vi "ExpXpecParser.vi"() -> ()   [LabVIEW 2010]
uses:
  <vilib>/xml/NI_XML.lvlib
panel:
  out "error in (no error)":errorcluster
  out "CSG 2":csg caption="CSG"
  out "CDB 2":cdb caption="CDB"
  out "CXT 2":cxt caption="CXT"
  out "U 65":u64 caption="U 64"
  out "U 33":u32 caption="U 32"
  out "U 17":u16 caption="U 16"
  out "I 9":i64 caption="I 8"
  out "I 65":i64 caption="I 64"
  out "EXT 2":ext caption="EXT"
  out "I16 2":i16
  out "FXP 2":fxp<+,1,1> caption="FXP"
  out "Single 2":sgl
  out "I 33":i32 caption="I 32"
  out "U 9":i32 caption="U 8"
  out "String 2":string caption="String"
  out "Double 2":dbl caption="Double"
  out "parse errors":string
  in  "Root in":string="/experimentSpecification/terminal/function/"
  in  "input array":variant[](array[variant])
  out "XML-String-in":string
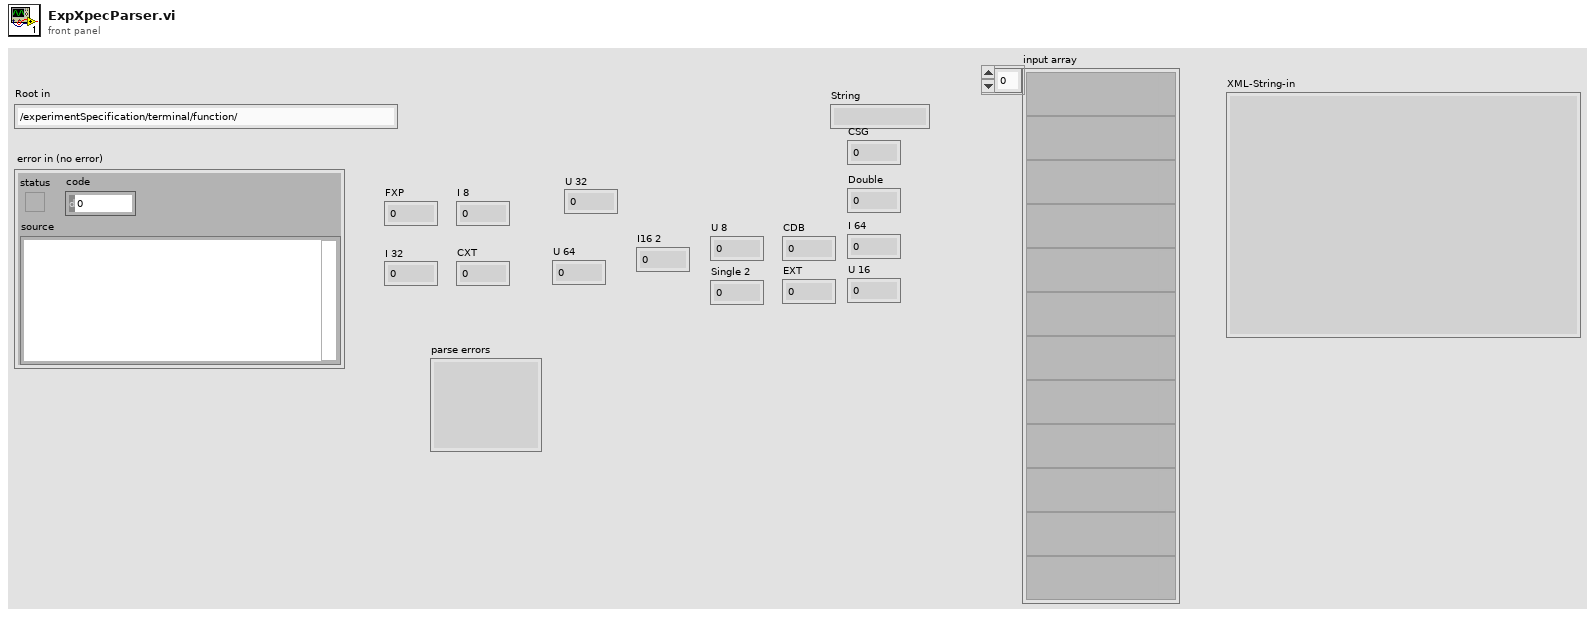
[diagram p1: front panel]
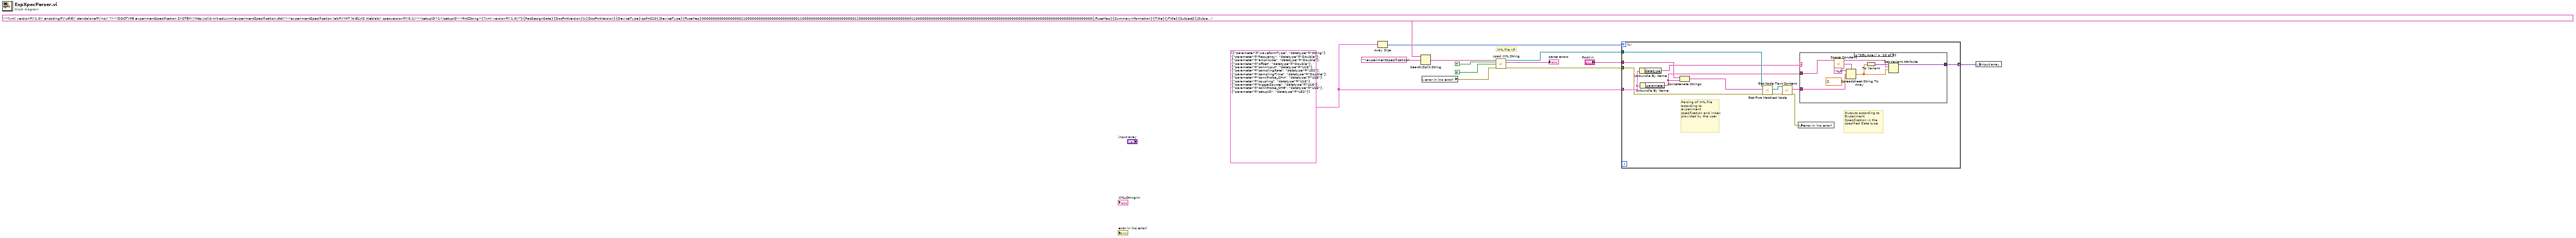
[diagram p0: block diagram]
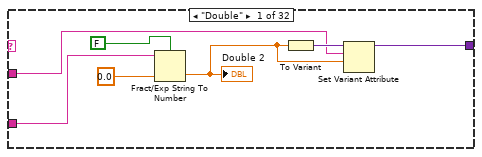
[diagram p2: hidden frame]
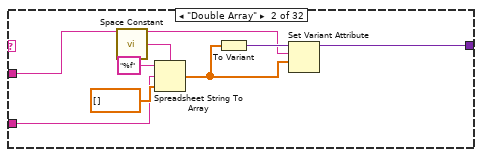
[diagram p3: hidden frame]
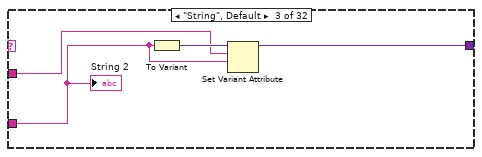
[diagram p4: hidden frame]
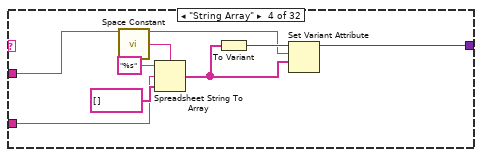
[diagram p5: hidden frame]
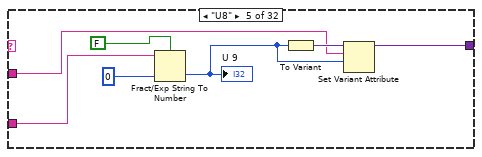
[diagram p6: hidden frame]
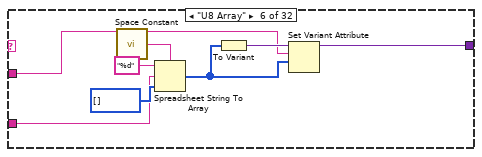
[diagram p7: hidden frame]
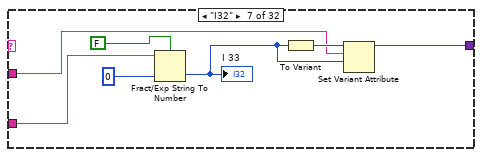
[diagram p8: hidden frame]
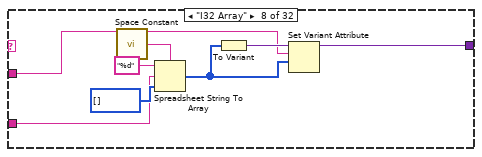
[diagram p9: hidden frame]
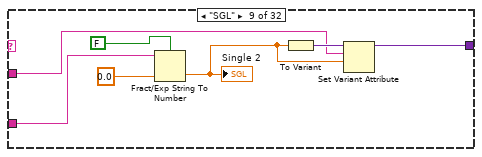
[diagram p10: hidden frame]
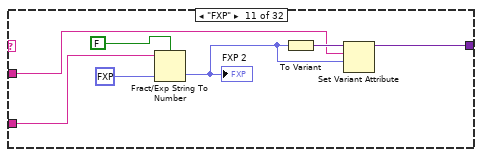
[diagram p11: hidden frame]
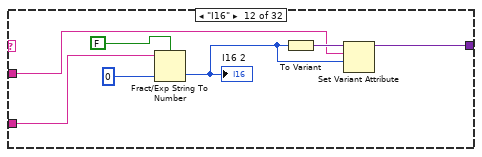
[diagram p12: hidden frame]
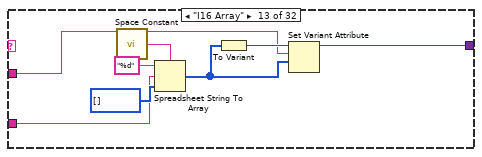
[diagram p13: hidden frame]
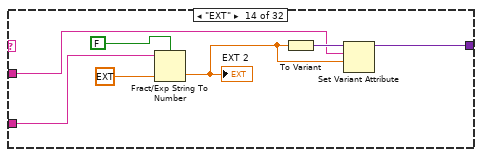
[diagram p14: hidden frame]
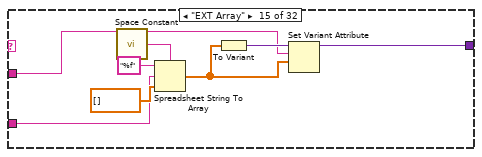
[diagram p15: hidden frame]
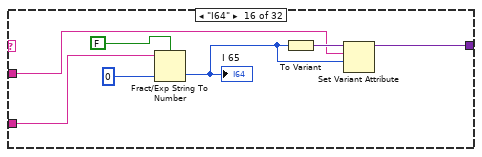
[diagram p16: hidden frame]
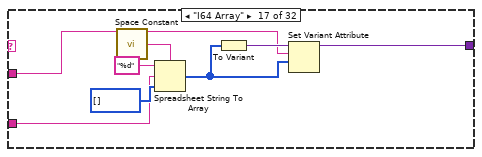
[diagram p17: hidden frame]
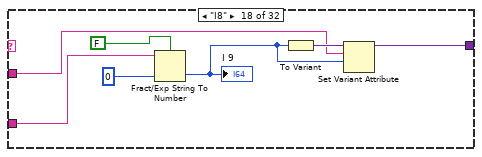
[diagram p18: hidden frame]
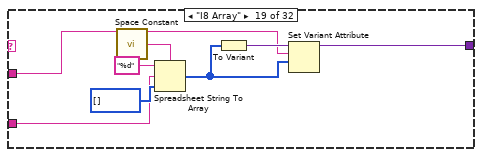
[diagram p19: hidden frame]
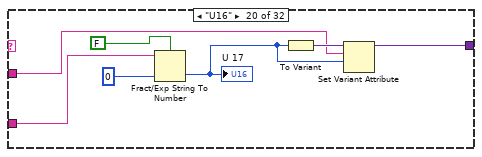
[diagram p20: hidden frame]
diagram:
  w3 = cluster{"parameter":string, "datatype":string}[] [{"parameter"="waveformType", "datatype"="String"}, {"parameter"="frequency", "datatype"="Double"}, {"parameter"="amplitude", "datatype"="Double"}, {"parameter"="offset", "datatype"="Double"}, {"parameter"="connInput", "datatype"="U16"}, {"parameter"="samplingRate", "datatype"="U32"}, {"parameter"="samplingTime", "datatype"="Double"}, {"parameter"="connProbe_CHA", "datatype"="U16"}, {"parameter"="coupling", "datatype"="U16"}, {"parameter"="triggerSource", "datatype"="U16"}, {"parameter"="connProbe_CHB", "datatype"="U16"}, {"parameter"="setupID", "datatype"="U32"}] ("Parameter in")
  # "XML file I/P"
  n1 = Array Size(array=w3) -> (size(s)=w1:i32)
  n2 = Search/Split String(string="<?xml version=\"1.0\" encoding=\"utf-8\" standalone=\"no\" ?><!DOCTYPE experimentSpecification SYSTEM \"http://olid.mit.edu/xml/experimentSpecification.dtd\"><experimentSpecification lab=\"MIT NI-ELVIS Weblab\" specversion=\"0.1\"><setupID>1</setupID><PACString>{?xml version=\"1.0\"?}{PacDesignData}{DocFmtVersion}1{/DocFmtVersion}{DeviceType}ispPAC10{/DeviceType}{FuseMap}00000000000000000011000000000000000000000000110000000000000000000000001100000000000000000000000011000000000000000000000000000000000000000000000000000000000000000000000000000000000{/FuseMap}{SummaryInformation}{Title}{/Title}{Subject}{/Subject}{Author}CTI{/Author}{Keywords}ispPAC10{/Keywords}{Comments}{![CDATA[]]}{/Comments}{/SummaryInformation}{/PacDesignData}</PACString><terminal instrumentType=\"FGEN\" instrumentNumber=\"1\"><vname download=\"true\">Vin</vname><function type=\"WAVEFORM\"><waveformType>SINE</waveformType><frequency>100.0</frequency><amplitude>1.0</amplitude><offset>5.0</offset><connInput>0</connInput></function></terminal><terminal instrumentType=\"SCOPE\" instrumentNumber=\"2\"><vname download=\"true\">Vout</vname><function type=\"SAMPLING\"><samplingRate>100000</samplingRate><samplingTime>0.01</samplingTime><connProbe_CHA>0</connProbe_CHA><coupling>1</coupling><triggerSource>0</triggerSource><connProbe_CHB>0</connProbe_CHB></function></terminal></experimentSpecification>" ("XML-String-in"), search string/char (-)="<experimentSpecification") -> (match + rest of string=w4:string)  [unwired: 1 in, 2 out]
  n3 = local read "error in (no error)"() -> (w6:errorcluster)
  n4 = call <vilib>:"Load XML String.vi"("XML string"=w4, "process namespaces (False)"=TRUE, "process schema (False)"=FALSE, "error in (no error)"=w6) -> ("DOM document out"=w9:refnum<k20>, "parse errors"=→"parse errors":string, "error out"=w10:errorcluster)  [unwired: 9 out]
  n5 = for {
    N: w1 -> [_]
    tunnel: w9 -> [w25]
    tunnel: "Root in" -> [w22]
    tunnel: w3 -> [w20] mode=indexing
    tunnel: w10 -> [w19]
    tunnel: [w18] -> w7 mode=indexing
    # "Outputs according to Experiment Specification in the specified Data type"
    # "Parsing of XML file according to experiment specification and index provided by the user"
    n6 = Unbundle By Name(w20) -> ("datatype"=w17:string)
    n7 = Unbundle By Name(w20) -> ("parameter"=w15:string)
    n8 = Concatenate Strings(w22, w15) -> (w21:string)
    n9 = call <vilib>:"Get First Matched Node.vi"("error in (no error)"=w19, "XPath expression"=w21, "node in"=w25) -> ("error out"=w23:errorcluster, "node result"=w24:refnum<k20>)  [unwired: 6 in, 1 out]
    n10 = call <vilib>:"Get Node Text Content.vi"("error in (no error)"=w23, "node in"=w24) -> ("error out"=w14:errorcluster, "node text"=w16:string)  [unwired: 7 in, 1 out]
    n11 = local write "error in (no error)"(w14) -> ()
    n12 = case shown="\"SGL Array\"" w17 {
      tunnel: w15 -> [w26 w34 w41 w45 w53 w60 w68 w76 w83 w91 w98 w105 w112 w120 w128 w135 w142 w150 w157 w165 w172 w180 w187 w195 w202 w210 w218 w226 w233 w240 w248 w255]
      tunnel: w16 -> [w27 w33 w42 w46 w54 w61 w69 w75 w84 w90 w99 w106 w113 w121 w127 w136 w143 w151 w158 w166 w173 w181 w188 w196 w203 w211 w217 w225 w232 w241 w247 w256]
      tunnel: [w29 w36 w43 w49 w56 w64 w71 w79 w86 w93 w101 w108 w116 w123 w130 w138 w146 w153 w161 w168 w176 w183 w191 w198 w206 w213 w220 w228 w235 w243 w250 w258] -> w18
      frame "Double" {
        n13 = Fract/Exp String To Number(use system decimal point (T)=FALSE, string=w27, default (0 dbl)=0.0) -> (number=w28:dbl)  [unwired: 1 in, 1 out]
        "Double 2" <- w28
        n14 = To Variant(anything=w28) -> (Variant=w30:variant)
        n15 = Set Variant Attribute(Variant=w30, name=w26, value=w28) -> (Variant out=w29:variant)  [unwired: 1 in, 2 out]
      }
      frame "Double Array" {
        n16 = call <vilib>:"Space Constant.vi"() -> ("String"=w38:string)
        n17 = Spreadsheet String To Array(delimiter (Tab)=w38, format string="%f", spreadsheet string=w33, array type (2D Dbl)=dbl[] [] ("Array")) -> (array=w35:dbl[])
        n18 = To Variant(anything=w35) -> (Variant=w37:variant)
        n19 = Set Variant Attribute(Variant=w37, name=w34, value=w35) -> (Variant out=w36:variant)  [unwired: 1 in, 2 out]
      }
      frame "String", Default {
        n20 = To Variant(anything=w42) -> (Variant=w44:variant)
        n21 = Set Variant Attribute(Variant=w44, name=w41, value=w42) -> (Variant out=w43:variant)  [unwired: 1 in, 2 out]
        "String 2" <- w42
      }
      frame "String Array" {
        n22 = call <vilib>:"Space Constant.vi"() -> ("String"=w51:string)
        n23 = Spreadsheet String To Array(delimiter (Tab)=w51, format string="%s", spreadsheet string=w46, array type (2D Dbl)=string[] [] ("Array")) -> (array=w48:string[])
        n24 = To Variant(anything=w48) -> (Variant=w50:variant)
        n25 = Set Variant Attribute(Variant=w50, name=w45, value=w48) -> (Variant out=w49:variant)  [unwired: 1 in, 2 out]
      }
      frame "U8" {
        n26 = Fract/Exp String To Number(use system decimal point (T)=FALSE, string=w54, default (0 dbl)=u8 0) -> (number=w55:u8)  [unwired: 1 in, 1 out]
        "U 9" <- w55
        n27 = To Variant(anything=w55) -> (Variant=w57:variant)
        n28 = Set Variant Attribute(Variant=w57, name=w53, value=w55) -> (Variant out=w56:variant)  [unwired: 1 in, 2 out]
      }
      frame "U8 Array" {
        n29 = call <vilib>:"Space Constant.vi"() -> ("String"=w66:string)
        n30 = Spreadsheet String To Array(delimiter (Tab)=w66, format string="%d", spreadsheet string=w61, array type (2D Dbl)=u8[] [] ("Array")) -> (array=w62:u8[])
        n31 = To Variant(anything=w62) -> (Variant=w65:variant)
        n32 = Set Variant Attribute(Variant=w65, name=w60, value=w62) -> (Variant out=w64:variant)  [unwired: 1 in, 2 out]
      }
      frame "I32" {
        n33 = Fract/Exp String To Number(use system decimal point (T)=FALSE, string=w69, default (0 dbl)=0) -> (number=w70:i32)  [unwired: 1 in, 1 out]
        "I 33" <- w70
        n34 = To Variant(anything=w70) -> (Variant=w72:variant)
        n35 = Set Variant Attribute(Variant=w72, name=w68, value=w70) -> (Variant out=w71:variant)  [unwired: 1 in, 2 out]
      }
      frame "I32 Array" {
        n36 = call <vilib>:"Space Constant.vi"() -> ("String"=w81:string)
        n37 = Spreadsheet String To Array(delimiter (Tab)=w81, format string="%d", spreadsheet string=w75, array type (2D Dbl)=i32[] [] ("Array")) -> (array=w77:i32[])
        n38 = To Variant(anything=w77) -> (Variant=w80:variant)
        n39 = Set Variant Attribute(Variant=w80, name=w76, value=w77) -> (Variant out=w79:variant)  [unwired: 1 in, 2 out]
      }
      frame "SGL" {
        n40 = Fract/Exp String To Number(use system decimal point (T)=FALSE, string=w84, default (0 dbl)=sgl 0.0) -> (number=w85:sgl)  [unwired: 1 in, 1 out]
        "Single 2" <- w85
        n41 = To Variant(anything=w85) -> (Variant=w87:variant)
        n42 = Set Variant Attribute(Variant=w87, name=w83, value=w85) -> (Variant out=w86:variant)  [unwired: 1 in, 2 out]
      }
      frame "SGL Array" {
        n43 = call <vilib>:"Space Constant.vi"() -> ("String"=w95:string)
        n44 = Spreadsheet String To Array(delimiter (Tab)=w95, format string="%f", spreadsheet string=w90, array type (2D Dbl)=sgl[] [] ("Array")) -> (array=w92:sgl[])
        n45 = To Variant(anything=w92) -> (Variant=w94:variant)
        n46 = Set Variant Attribute(Variant=w94, name=w91, value=w92) -> (Variant out=w93:variant)  [unwired: 1 in, 2 out]
      }
      frame "FXP" {
        n47 = Fract/Exp String To Number(use system decimal point (T)=FALSE, string=w99, default (0 dbl)=fxp<+,1,1> 0.0) -> (number=w100:fxp<+,1,1>)  [unwired: 1 in, 1 out]
        "FXP 2" <- w100
        n48 = To Variant(anything=w100) -> (Variant=w102:variant)
        n49 = Set Variant Attribute(Variant=w102, name=w98, value=w100) -> (Variant out=w101:variant)  [unwired: 1 in, 2 out]
      }
      frame "I16" {
        n50 = Fract/Exp String To Number(use system decimal point (T)=FALSE, string=w106, default (0 dbl)=i16 0 ("I16")) -> (number=w109:i16)  [unwired: 1 in, 1 out]
        "I16 2" <- w109
        n51 = To Variant(anything=w109) -> (Variant=w110:variant)
        n52 = Set Variant Attribute(Variant=w110, name=w105, value=w109) -> (Variant out=w108:variant)  [unwired: 1 in, 2 out]
      }
      frame "I16 Array" {
        n53 = call <vilib>:"Space Constant.vi"() -> ("String"=w118:string)
        n54 = Spreadsheet String To Array(delimiter (Tab)=w118, format string="%d", spreadsheet string=w113, array type (2D Dbl)=i16[] [] ("Array")) -> (array=w114:i16[])
        n55 = To Variant(anything=w114) -> (Variant=w117:variant)
        n56 = Set Variant Attribute(Variant=w117, name=w112, value=w114) -> (Variant out=w116:variant)  [unwired: 1 in, 2 out]
      }
      frame "EXT" {
        n57 = Fract/Exp String To Number(use system decimal point (T)=FALSE, string=w121, default (0 dbl)=ext 0.0) -> (number=w122:ext)  [unwired: 1 in, 1 out]
        "EXT 2" <- w122
        n58 = To Variant(anything=w122) -> (Variant=w124:variant)
        n59 = Set Variant Attribute(Variant=w124, name=w120, value=w122) -> (Variant out=w123:variant)  [unwired: 1 in, 2 out]
      }
      frame "EXT Array" {
        n60 = call <vilib>:"Space Constant.vi"() -> ("String"=w132:string)
        n61 = Spreadsheet String To Array(delimiter (Tab)=w132, format string="%f", spreadsheet string=w127, array type (2D Dbl)=ext[] [] ("Array")) -> (array=w129:ext[])
        n62 = To Variant(anything=w129) -> (Variant=w131:variant)
        n63 = Set Variant Attribute(Variant=w131, name=w128, value=w129) -> (Variant out=w130:variant)  [unwired: 1 in, 2 out]
      }
      frame "I64" {
        n64 = Fract/Exp String To Number(use system decimal point (T)=FALSE, string=w136, default (0 dbl)=i64 0) -> (number=w137:i64)  [unwired: 1 in, 1 out]
        "I 65" <- w137
        n65 = To Variant(anything=w137) -> (Variant=w139:variant)
        n66 = Set Variant Attribute(Variant=w139, name=w135, value=w137) -> (Variant out=w138:variant)  [unwired: 1 in, 2 out]
      }
      frame "I64 Array" {
        n67 = call <vilib>:"Space Constant.vi"() -> ("String"=w148:string)
        n68 = Spreadsheet String To Array(delimiter (Tab)=w148, format string="%d", spreadsheet string=w143, array type (2D Dbl)=i64[] [] ("Array")) -> (array=w144:i64[])
        n69 = To Variant(anything=w144) -> (Variant=w147:variant)
        n70 = Set Variant Attribute(Variant=w147, name=w142, value=w144) -> (Variant out=w146:variant)  [unwired: 1 in, 2 out]
      }
      frame "I8" {
        n71 = Fract/Exp String To Number(use system decimal point (T)=FALSE, string=w151, default (0 dbl)=i8 0) -> (number=w152:i8)  [unwired: 1 in, 1 out]
        "I 9" <- w152
        n72 = To Variant(anything=w152) -> (Variant=w154:variant)
        n73 = Set Variant Attribute(Variant=w154, name=w150, value=w152) -> (Variant out=w153:variant)  [unwired: 1 in, 2 out]
      }
      frame "I8 Array" {
        n74 = call <vilib>:"Space Constant.vi"() -> ("String"=w163:string)
        n75 = Spreadsheet String To Array(delimiter (Tab)=w163, format string="%d", spreadsheet string=w158, array type (2D Dbl)=i8[] [] ("Array")) -> (array=w159:i8[])
        n76 = To Variant(anything=w159) -> (Variant=w162:variant)
        n77 = Set Variant Attribute(Variant=w162, name=w157, value=w159) -> (Variant out=w161:variant)  [unwired: 1 in, 2 out]
      }
      frame "U16" {
        n78 = Fract/Exp String To Number(use system decimal point (T)=FALSE, string=w166, default (0 dbl)=u16 0) -> (number=w167:u16)  [unwired: 1 in, 1 out]
        "U 17" <- w167
        n79 = To Variant(anything=w167) -> (Variant=w169:variant)
        n80 = Set Variant Attribute(Variant=w169, name=w165, value=w167) -> (Variant out=w168:variant)  [unwired: 1 in, 2 out]
      }
      frame "U16 Array" {
        n81 = call <vilib>:"Space Constant.vi"() -> ("String"=w178:string)
        n82 = Spreadsheet String To Array(delimiter (Tab)=w178, format string="%d", spreadsheet string=w173, array type (2D Dbl)=u16[] [] ("Array")) -> (array=w174:u16[])
        n83 = To Variant(anything=w174) -> (Variant=w177:variant)
        n84 = Set Variant Attribute(Variant=w177, name=w172, value=w174) -> (Variant out=w176:variant)  [unwired: 1 in, 2 out]
      }
      frame "U32" {
        n85 = Fract/Exp String To Number(use system decimal point (T)=FALSE, string=w181, default (0 dbl)=u32 0) -> (number=w182:u32)  [unwired: 1 in, 1 out]
        "U 33" <- w182
        n86 = To Variant(anything=w182) -> (Variant=w184:variant)
        n87 = Set Variant Attribute(Variant=w184, name=w180, value=w182) -> (Variant out=w183:variant)  [unwired: 1 in, 2 out]
      }
      frame "U32 Array" {
        n88 = call <vilib>:"Space Constant.vi"() -> ("String"=w193:string)
        n89 = Spreadsheet String To Array(delimiter (Tab)=w193, format string="%d", spreadsheet string=w188, array type (2D Dbl)=u32[] [] ("Array")) -> (array=w189:u32[])
        n90 = To Variant(anything=w189) -> (Variant=w192:variant)
        n91 = Set Variant Attribute(Variant=w192, name=w187, value=w189) -> (Variant out=w191:variant)  [unwired: 1 in, 2 out]
      }
      frame "U64" {
        n92 = Fract/Exp String To Number(use system decimal point (T)=FALSE, string=w196, default (0 dbl)=u64 0) -> (number=w197:u64)  [unwired: 1 in, 1 out]
        "U 65" <- w197
        n93 = To Variant(anything=w197) -> (Variant=w199:variant)
        n94 = Set Variant Attribute(Variant=w199, name=w195, value=w197) -> (Variant out=w198:variant)  [unwired: 1 in, 2 out]
      }
      frame "U64 Array" {
        n95 = call <vilib>:"Space Constant.vi"() -> ("String"=w208:string)
        n96 = Spreadsheet String To Array(delimiter (Tab)=w208, format string="%d", spreadsheet string=w203, array type (2D Dbl)=u64[] [] ("Array")) -> (array=w204:u64[])
        n97 = To Variant(anything=w204) -> (Variant=w207:variant)
        n98 = Set Variant Attribute(Variant=w207, name=w202, value=w204) -> (Variant out=w206:variant)  [unwired: 1 in, 2 out]
      }
      frame "CXT" {
        n99 = Scan From String(format string="%f", input string=w211, default 1=cxt 0.0+0.0i ("number 3")) -> (output 1=w212:cxt)  [unwired: 2 in, 3 out]
        "CXT 2" <- w212
        n100 = To Variant(anything=w212) -> (Variant=w214:variant)
        n101 = Set Variant Attribute(Variant=w214, name=w210, value=w212) -> (Variant out=w213:variant)  [unwired: 1 in, 2 out]
      }
      frame "CXT Array" {
        n102 = call <vilib>:"Space Constant.vi"() -> ("String"=w222:string)
        n103 = Spreadsheet String To Array(delimiter (Tab)=w222, format string="%f", spreadsheet string=w217, array type (2D Dbl)=cxt[] [] ("Array")) -> (array=w219:cxt[])
        n104 = To Variant(anything=w219) -> (Variant=w221:variant)
        n105 = Set Variant Attribute(Variant=w221, name=w218, value=w219) -> (Variant out=w220:variant)  [unwired: 1 in, 2 out]
      }
      frame "CDB" {
        n106 = Scan From String(format string="%f", input string=w225, default 1=cdb 0.0+0.0i ("number 3")) -> (output 1=w227:cdb)  [unwired: 2 in, 3 out]
        "CDB 2" <- w227
        n107 = To Variant(anything=w227) -> (Variant=w229:variant)
        n108 = Set Variant Attribute(Variant=w229, name=w226, value=w227) -> (Variant out=w228:variant)  [unwired: 1 in, 2 out]
      }
      frame "CDB Array" {
        n109 = call <vilib>:"Space Constant.vi"() -> ("String"=w237:string)
        n110 = Spreadsheet String To Array(delimiter (Tab)=w237, format string="%f", spreadsheet string=w232, array type (2D Dbl)=cdb[] [] ("Array")) -> (array=w234:cdb[])
        n111 = To Variant(anything=w234) -> (Variant=w236:variant)
        n112 = Set Variant Attribute(Variant=w236, name=w233, value=w234) -> (Variant out=w235:variant)  [unwired: 1 in, 2 out]
      }
      frame "CSG" {
        n113 = Scan From String(format string="%f", input string=w241, default 1=csg 0.0+0.0i ("number 3")) -> (output 1=w242:csg)  [unwired: 2 in, 3 out]
        "CSG 2" <- w242
        n114 = To Variant(anything=w242) -> (Variant=w244:variant)
        n115 = Set Variant Attribute(Variant=w244, name=w240, value=w242) -> (Variant out=w243:variant)  [unwired: 1 in, 2 out]
      }
      frame "CSG Array" {
        n116 = call <vilib>:"Space Constant.vi"() -> ("String"=w252:string)
        n117 = Spreadsheet String To Array(delimiter (Tab)=w252, format string="%f", spreadsheet string=w247, array type (2D Dbl)=csg[] [] ("Array")) -> (array=w249:csg[])
        n118 = To Variant(anything=w249) -> (Variant=w251:variant)
        n119 = Set Variant Attribute(Variant=w251, name=w248, value=w249) -> (Variant out=w250:variant)  [unwired: 1 in, 2 out]
      }
      frame "Boolean" {
        n120 = case shown="\"False\", Default" w256 {
          tunnel: [FALSE TRUE TRUE FALSE TRUE FALSE TRUE FALSE] -> w257
          frame "False", Default {
          }
          frame "True" {
          }
          frame "TRUE" {
          }
          frame "FALSE" {
          }
          frame "1" {
          }
          frame "0" {
          }
          frame "true" {
          }
          frame "false" {
          }
        }
        n121 = To Variant(anything=w257) -> (Variant=w259:variant)
        n122 = Set Variant Attribute(Variant=w259, name=w255, value=w257) -> (Variant out=w258:variant)  [unwired: 1 in, 2 out]
      }
    }
  }
  n123 = local write "input array"(w7) -> ()
